vi "build_jki_flat_icons_path.vi"(8 "error in (no error)":errorcluster) -> (0 "error out":errorcluster, 3 "jki flat icon path":path)   [LabVIEW 2020]
uses:
  <vilib>/Utility/sysdir.llb/System Directory Type.ctl
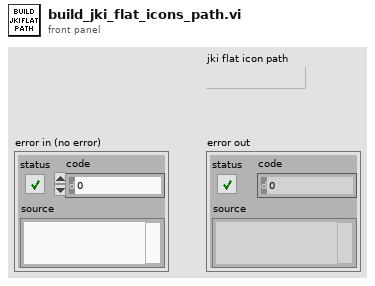
[diagram p1: front panel]
types:
  T1 = typedef "System Directory Type.ctl" = i32
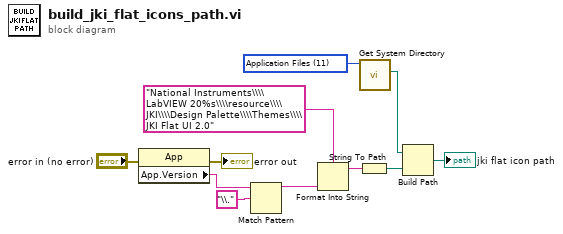
[diagram p0: block diagram]
diagram:
  w2 = T1 11 items=["User Home"=0, "User Desktop"=1, "User Documents"=2, "User Application Data"=3, "User Preferences"=4, "User Temporary"=5, "Public Documents"=6, "Public Application Data"=7, "Public Preferences"=8, "Public Cache"=13, "System Core Libraries"=9, "System Installed Libraries"=10, "Application Files"=11, "Boot Volume Root"=12] ("system directory type")
  n1 = property class="App"(error in="error in (no error)") -> (error out=→"error out":errorcluster, "App.Version"=w8:string)  [unwired: 1 in, 1 out]
  n2 = Match Pattern(string=w8, regular expression="\\.") -> (before substring=w5:string)  [unwired: 1 in, 3 out]
  n3 = Format Into String(format string="National Instruments\\\\LabVIEW 20%s\\\\resource\\\\JKI\\\\Design Palette\\\\Themes\\\\JKI Flat UI 2.0", w5) -> (resulting string=w7:string)  [unwired: 2 in, 1 out]
  n4 = String To Path(string=w7) -> (path=w10:path)
  n5 = call <vilib>:"Get System Directory.vi"("system directory type"=w2) -> ("system directory"=w1:path)  [unwired: 10 in]
  n6 = Build Path(base path=w1, name or relative path=w10) -> (appended path=→"jki flat icon path":path)
